vi "Open SQL Connection.vi"(8 "error in (no error)":errorcluster, 10 "SQL Data":variant, 11 "SQLObject in":refnum<class "SQLObject.lvclass">) -> (0 "error out":errorcluster, 2 "Boolean":bool, 3 "SQLObject out":refnum<class "SQLObject.lvclass">)   [LabVIEW 2021, in "SQLObject.lvclass"]
uses:
  SQLObject.lvclass
  SQLObject.lvclass/SQLObject.ctl
  <vilib>/drjdpowell/SQLite Library/SQL Connection/Open (path).vi
  <vilib>/drjdpowell/SQLite Library/SQL Connection/Open (string).vi
  <vilib>/AdvancedString/Path To Command Line String.vi
  <vilib>/drjdpowell/SQLite Library/SQL Connection/Execute SQL (Single String).vi
  <vilib>/drjdpowell/SQLite Library/SQL Connection/Connection.lvclass
  <vilib>/drjdpowell/SQLite Library/SQLite.lvlib
  <vilib>/Utility/Data Type/NI_Data Type.lvlib
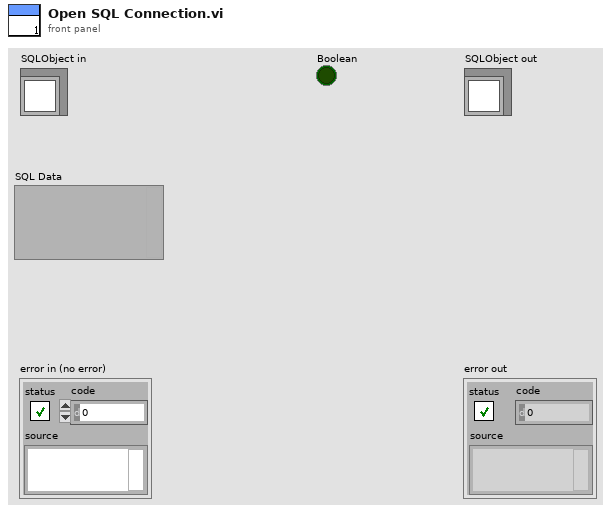
[diagram p1: front panel]
types:
  T1 = enum16{"New or existing", "Existing", "Read only"}
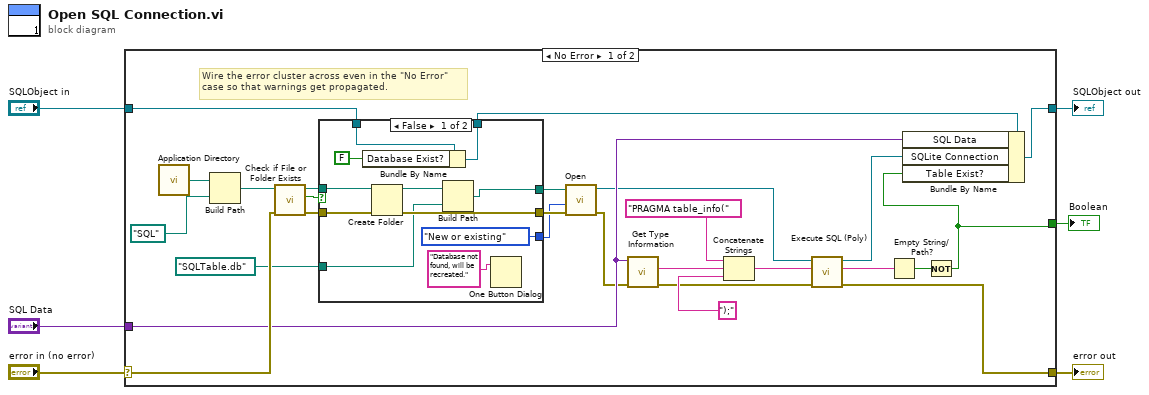
[diagram p0: block diagram]
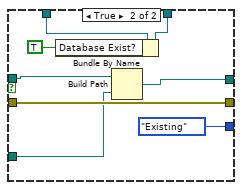
[diagram p2: hidden frame]
diagram:
  n1 = case shown="No Error" "error in (no error)" {
    selector: "error in (no error)" -> [w30 w54]
    tunnel: [w10 w54] -> w5
    tunnel: [w22 w53] -> w3
    tunnel: "SQLObject in" -> [w28 w53]
    tunnel: "SQL Data" -> [w18 _]
    tunnel: [w7 _] -> w1
    frame No Error {
      # "Wire the error cluster across even in the \"No Error\"\ncase so that warnings get propagated."
      n2 = call <vilib>:"Application Directory.vi"() -> ("Application Directory"=w33:path)
      n3 = Build Path(base path=w33, name or relative path=path "SQL") -> (appended path=w32:path)
      n4 = call <vilib>:"Check if File or Folder Exists.vi"("error in (no error)"=w30, "path"=w32) -> ("error out"=w26:errorcluster, "file or folder exists?"=w29:bool, "dup path"=w27:path)  [unwired: 7 in]
      n5 = case shown="False" w29 {
        tunnel: w28 -> [w44 w51]
        tunnel: w27 -> [w43 w49]
        tunnel: [w41 w50] -> w23
        tunnel: w26 -> [w40 w48]
        tunnel: [w37 w47] -> w25
        tunnel: [w39 w48] -> w24
        tunnel: [T1."New or existing" ("File Option") T1."Existing" ("File Option")] -> w21
        tunnel: path "SQLTable.db" ("name or relative path") -> [w34 w45]
        frame False {
          n6 = Bundle By Name(cluster=w44, "Database Exist?"=FALSE ("SQL Folder Exist?")) -> (w41:refnum<class "SQLObject.lvclass">)
          n7 = Create Folder(path (use dialog)=w43, error in=w40) -> (created path=w38:path, error out=w39:errorcluster)  [unwired: 1 in, 1 out]
          n8 = Build Path(base path=w38, name or relative path=w34) -> (appended path=w37:path)
          n9 = One Button Dialog(message="Database not found, will be recreated.") -> ()  [unwired: 1 in, 1 out]
        }
        frame True {
          n10 = Bundle By Name(cluster=w51, "Database Exist?"=TRUE ("SQL Folder Exist?")) -> (w50:refnum<class "SQLObject.lvclass">)
          n11 = Build Path(base path=w49, name or relative path=w45) -> (appended path=w47:path)
        }
      }
      n12 = call-poly <vilib>:"Open.vi"("error in (no error)"=w24, "File Option"=w21, "db file"=w25) -> ("error out"=w17:errorcluster, "SQLite Connection"=w13:refnum<class "Connection.lvclass">)  [unwired: 7 in]
      n13 = call <vilib>:"Get Type Information.vi"("error in (no error)"=w17, "variant"=w18) -> ("error out"=w11:errorcluster, "name"=w15:string)  [unwired: 5 in, 3 out]
      n14 = Concatenate Strings("PRAGMA table_info(" ("string"), w15, ");" ("string")) -> (w14:string)
      n15 = call-poly <vilib>:"Execute SQL (Poly).vi"("error in (no error)"=w11, "SQL"=w14, "SQLite Connection in"=w13) -> ("error out"=w10:errorcluster, "Result"=w16:string, "SQLite Connection"=w8:refnum<class "Connection.lvclass">)  [unwired: 6 in]
      n16 = Empty String/Path?(string/path=w16) -> (empty?=w12:bool)
      n17 = Not(x=w12) -> (.not. x?=w7:bool)
      n18 = Bundle By Name(cluster=w23, "SQL Data"=w18, "SQLite Connection"=w8, "Table Exist?"=w7) -> (w22:refnum<class "SQLObject.lvclass">)
    }
    frame Error {
    }
  }
  "error out" <- w5
  "SQLObject out" <- w3
  "Boolean" <- w1
